vi "PolishVisionV2.vi"() -> (0 "Vison Status":bool, 3 "Image Out":T1)   [LabVIEW 2015]
uses:
  <vilib>/vision/Image Controls.llb/IMAQ Image.ctl
  <vilib>/userdefined/High Color/IMAQdx.ctl
  <vilib>/vision/Pattern Matching.llb/IMAQ Curve Parameters.ctl
  <vilib>/vision/Pattern Matching.llb/IMAQ Match Range Setting.ctl
  <vilib>/vision/driver/NI_Vision_Acquisition_Software.lvlib
  <vilib>/vision/NI_Vision_Development_Module.lvlib
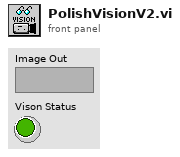
[diagram p1: front panel]
types:
  T1 = typedef "IMAQ Image.ctl" = refnum<image>
  T2 = typedef "IMAQdx.ctl" = refnum<k21>
  T3 = typedef "Image Type" = u32
  T4 = cluster{"Origin Pixel":cluster{"X":sgl, "Y":sgl}, "X Axis Pixel":cluster{"X":sgl, "Y":sgl}, "Axis Reference":u32}
  T5 = cluster{"Position":cluster{"X":sgl, "Y":sgl}, "Radius":dbl, "Score":dbl}[]
  T6 = cluster{"Circles[0]":cluster{"Position":cluster{"X":sgl, "Y":sgl}, "Radius":dbl, "Score":dbl}, "Circles[1]":cluster{"Position":cluster{"X":sgl, "Y":sgl}, "Radius":dbl, "Score":dbl}, "Circles[2]":cluster{"Position":cluster{"X":sgl, "Y":sgl}, "Radius":dbl, "Score":dbl}, "Circles[3]":cluster{"Position":cluster{"X":sgl, "Y":sgl}, "Radius":dbl, "Score":dbl}, "Circles[4]":cluster{"Position":cluster{"X":sgl, "Y":sgl}, "Radius":dbl, "Score":dbl}, "Circles[5]":cluster{"Position":cluster{"X":sgl, "Y":sgl}, "Radius":dbl, "Score":dbl}, "Circles[6]":cluster{"Position":cluster{"X":sgl, "Y":sgl}, "Radius":dbl, "Score":dbl}, "Circles[7]":cluster{"Position":cluster{"X":sgl, "Y":sgl}, "Radius":dbl, "Score":dbl}, "Circles[8]":cluster{"Position":cluster{"X":sgl, "Y":sgl}, "Radius":dbl, "Score":dbl}}
  T7 = typedef "IMAQ Curve Parameters.ctl" = cluster{"Extraction Mode":u32, "Edge Threshold":i32, "Edge Filter Size":u32, "Min Length":i32, "Row Search Step Size":i32, "Col Search Step Size":i32, "Max Endpoint Gap":i32, "Closed":bool, "Subpixel":bool}
  T8 = typedef "IMAQ Match Range Setting.ctl" = cluster{"Match Constraints":u32, "Min":dbl, "Max":dbl}
  T9 = cluster{"Curve Parameters":T7, "Match Mode":cluster{"Rotation":bool, "Scale":bool, "Occlusion":bool, "Reserved":bool, "Reserved":bool, "Reserved":bool}, "Range Settings":T8[], "Number of Matches":i32, "Minimum Match Score":sgl, "SubPixel Accuracy":bool, "Adv. Geometric Match Options 2":cluster{"Setup Data Item":u16, "Item Value":dbl}[]}
  T10 = cluster{"Global Rectangle":i32[], "Contours":cluster{"ID":enum32{"External", "Internal"}, "Type":u32, "Coordinates":i32[]}[]}
  T11 = typedef "IMAQ GM Match Report.ctl" = cluster{"Position":cluster{"x":sgl, "y":sgl}, "Angle":sgl, "Scale":sgl, "Score":sgl, "Bounding Box":cluster{"x":sgl, "y":sgl}[], "Contrast Reversed":bool, "Occlusion %":sgl, "Template Target Curve Score":sgl, "Target Template Curve Score":sgl, "Correlation Score":sgl}
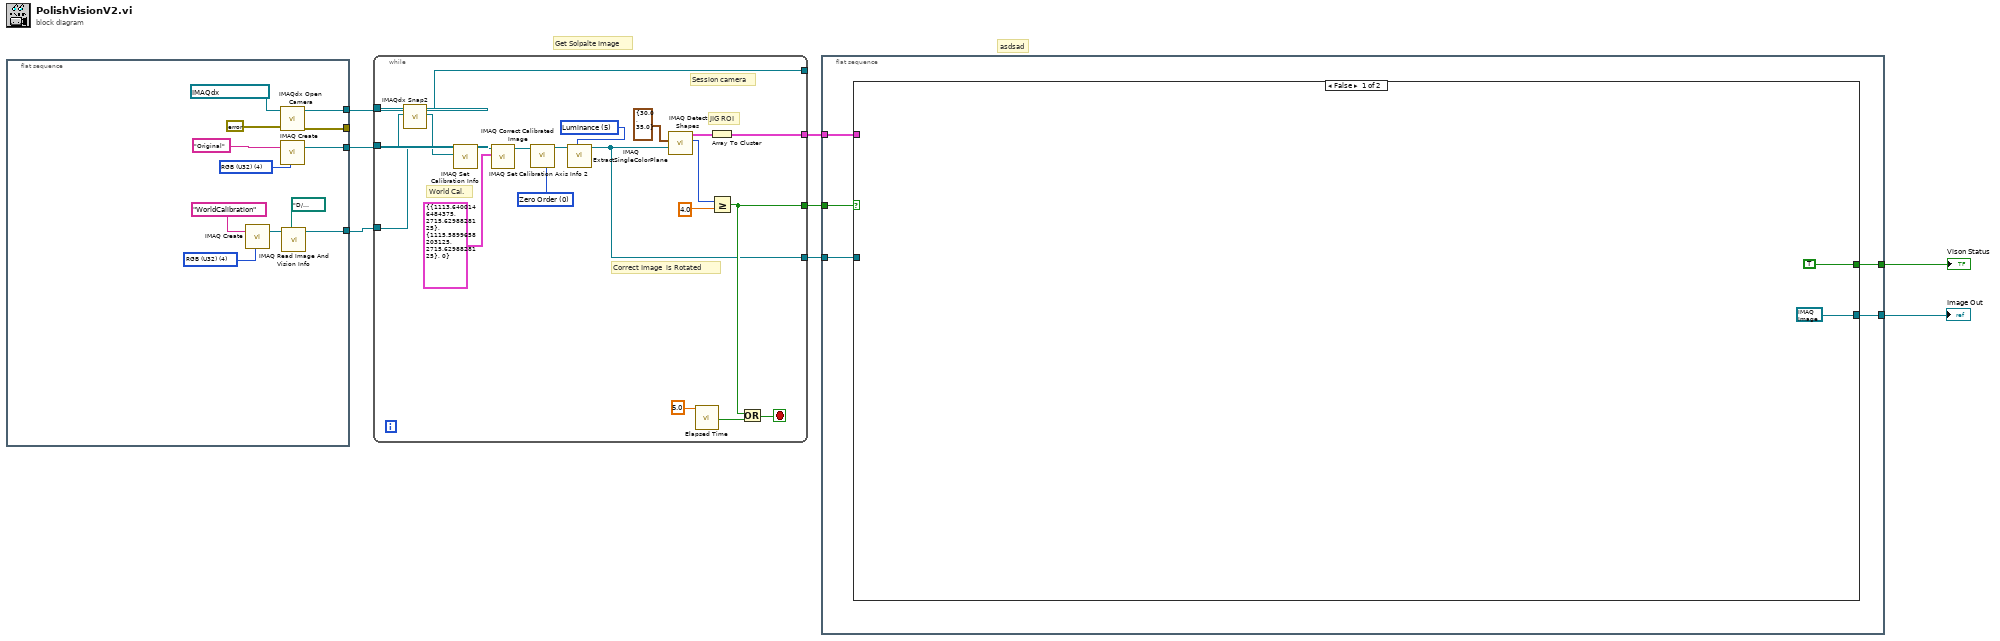
[diagram p0: block diagram]
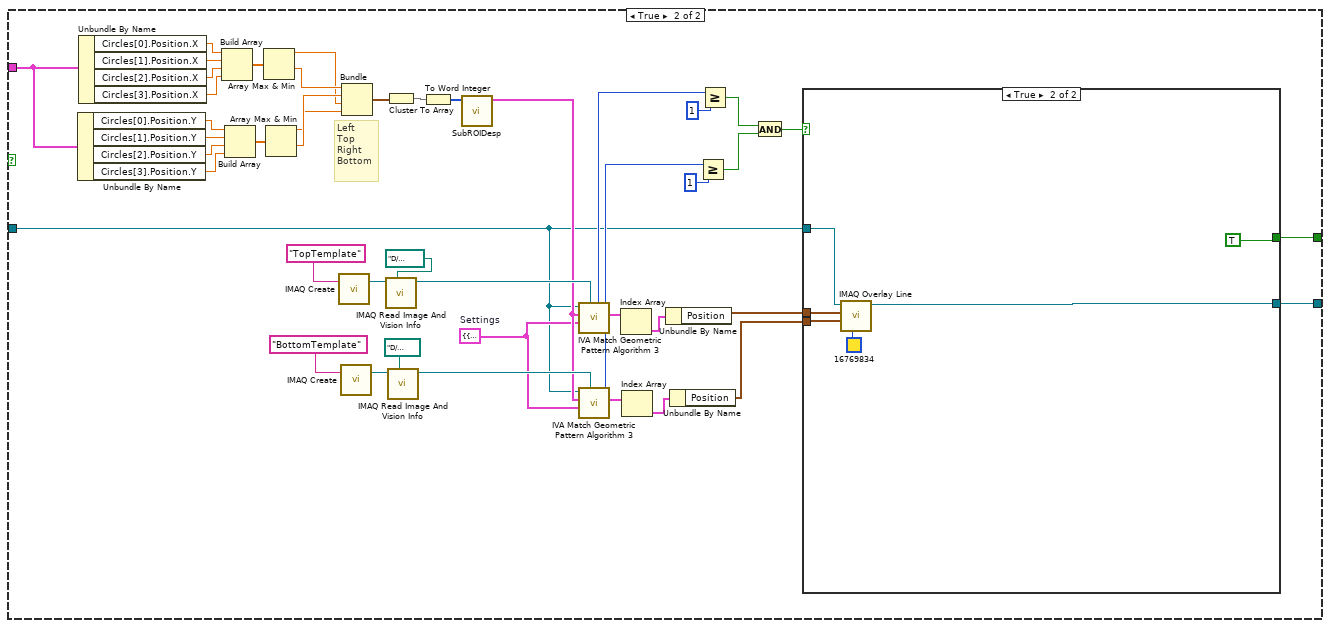
[diagram p2: hidden frame]
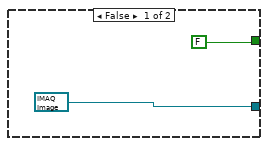
[diagram p3: hidden frame]
diagram:
  # "Get Solpalte Image"
  # "asdsad"
  n1 = flat-sequence {
    tunnel: [w17] -> w8
    tunnel: [w16] -> w7
    tunnel: [w15] -> _
    tunnel: [w10] -> w6
    frame #0 {
      w14 = T3 4 items=["Grayscale (U8)", "Grayscale (I16)", "Grayscale (SGL)", "Complex (CSG)", "RGB (U32)", "HSL (U32)", "RGB (U64)", "Grayscale (U16)"] ("Image Type")
      w18 = T3 4 items=["Grayscale (U8)", "Grayscale (I16)", "Grayscale (SGL)", "Complex (CSG)", "RGB (U32)", "HSL (U32)", "RGB (U64)", "Grayscale (U16)"] ("Image Type")
      n2 = call "IMAQ Create"("Image Name"="WorldCalibration", "Image Type"=w14) -> ("New Image"=w12:T1)  [unwired: 2 in, 2 out]
      n3 = call <vilib>:"IMAQdx Open Camera.vi"("error in"=errorcluster {"status"=FALSE, "code"=0, "source"=""}, "Session In"=T2 "RobotPolishCAM") -> ("error out"=w15:errorcluster, "Session Out"=w17:T2)  [unwired: 8 in]
      n4 = call "IMAQ Create"("Image Name"="Original", "Image Type"=w18) -> ("New Image"=w16:T1)  [unwired: 3 in, 1 out]
      n5 = call "IMAQ Read Image And Vision Info"("File Path"=path "D:/PolishingRobot/LastEdition/config setting/WorldCalV2.png", "Image"=w12) -> ("Image Out"=w10:T1)  [unwired: 2 in, 7 out]
    }
  }
  n6 = while {
    tunnel: w8 -> [w41]
    tunnel: w7 -> [w40]
    tunnel: [w28] -> w5
    tunnel: [w34] -> _
    tunnel: w6 -> [w22]
    tunnel: [w24] -> w4
    tunnel: [w23] -> w3
    stop <- w25 stop-if-true
    w31 = u32 0 items=["Zero Order", "Bi-Linear", "Quadratic", "Cubic Spline"] ("Interpolation Type")
    w39 = 5 items=["Red", "Green", "Blue", "Hue", "Saturation", "Luminance", "Value", "Intensity"] ("Color Plane")
    # "Correct Image  is Rotated"
    # "Session camera"
    # "World Cal."
    # "JIG ROI"
    n7 = call <vilib>:"IMAQdx Snap2.vi"("Image In"=w40, "Session In"=w41) -> ("Image Out"=w21:T1, "Session Out"=w34:T2)  [unwired: 7 in, 1 out]
    n8 = call "IMAQ Set Calibration Info"("Image Dst"=w21, "Image Src"=w22) -> ("Calibrated Image"=w32:T1)  [unwired: 2 in, 7 out]
    n9 = call-poly "IMAQ Set Calibration Axis Info 2"("Calibration Axis Info"=T4 {"Origin Pixel"={"X"=1113.64, "Y"=2715.63}, "X Axis Pixel"={"X"=1115.59, "Y"=2715.63}, "Axis Reference"=0}, "Calibration Template Image In"=w32) -> ("Calibration Template Image Out"=w30:T1)  [unwired: 1 in, 8 out]
    n10 = call "IMAQ Correct Calibrated Image"("Interpolation Type"=w31, "Image Src"=w30) -> ("Corrected Image"=w29:T1)  [unwired: 5 in, 4 out]
    n11 = call "IMAQ ExtractSingleColorPlane"("Color Plane"=w39, "Image Src"=w29) -> ("Image Dst Out"=w23:T1)  [unwired: 8 in, 1 out]
    n12 = call-poly "IMAQ Detect Shapes"("Circle Descriptor"=cluster{"Min Radius":dbl, "Max Radius":dbl} {"Min Radius"=30.0, "Max Radius"=35.0}, "Image"=w23) -> ("Number of Matches Returned"=w35:i32, "Circles"=w36:T5)  [unwired: 7 in, 1 out]
    n13 = call "Elapsed Time"("Time Target (s)"=5.0) -> ("Time has Elapsed"=w26:bool)  [unwired: 11 in, 7 out]
    n14 = Array To Cluster(array=w36) -> (cluster=w28:T6)
    n15 = Greater Or Equal?(x=w35, y=4.0) -> (x >= y?=w24:bool)
    n16 = Or(x=w24, y=w26) -> (x .or. y?=w25:bool)
  }
  n17 = flat-sequence {
    tunnel: w5 -> [w44]
    tunnel: w4 -> [w46]
    tunnel: w3 -> [w45]
    tunnel: [w43] -> w2
    tunnel: [w42] -> w1
    frame #0 {
      n18 = case shown="False" w46 {
        tunnel: w45 -> [_ w51]
        tunnel: w44 -> [_ w75]
        tunnel: [T1 refnum ("Image Out 2") w50] -> w43
        tunnel: [TRUE w49] -> w42
        frame False {
        }
        frame True {
          w65 = T9 {"Curve Parameters"={"Extraction Mode"=0, "Edge Threshold"=80, "Edge Filter Size"=1, "Min Length"=30, "Row Search Step Size"=10, "Col Search Step Size"=10, "Max Endpoint Gap"=10, "Closed"=FALSE, "Subpixel"=FALSE}, "Match Mode"={"Rotation"=TRUE, "Scale"=FALSE, "Occlusion"=FALSE, "Reserved"=FALSE, "Reserved"=FALSE, "Reserved"=FALSE}, "Range Settings"=[{"Match Constraints"=0, "Min"=-10.0, "Max"=10.0}], "Number of Matches"=1, "Minimum Match Score"=800.0, "SubPixel Accuracy"=FALSE, "Adv. Geometric Match Options 2"=[{"Setup Data Item"=21, "Item Value"=0.0}, {"Setup Data Item"=22, "Item Value"=1.0}]}  # Settings
          # "Left \nTop\nRight \nBottom"
          n19 = Unbundle By Name(w75) -> ("Circles[0].Position.Y"=w80:sgl, "Circles[1].Position.Y"=w79:sgl, "Circles[2].Position.Y"=w78:sgl, "Circles[3].Position.Y"=w77:sgl)
          n20 = Unbundle By Name(w75) -> ("Circles[0].Position.X"=w84:sgl, "Circles[1].Position.X"=w83:sgl, "Circles[2].Position.X"=w82:sgl, "Circles[3].Position.X"=w81:sgl)
          n21 = Build Array(w84, w83, w82, w81) -> (w76:sgl[])
          n22 = Build Array(w80, w79, w78, w77) -> (w74:sgl[])
          n23 = Array Max & Min(array=w76) -> (max value=w71:sgl, min value=w73:sgl)  [unwired: 2 out]
          n24 = Array Max & Min(array=w74) -> (max value=w70:sgl, min value=w72:sgl)  [unwired: 2 out]
          n25 = call "IMAQ Create"("Image Name"="TopTemplate") -> ("New Image"=w91:T1)  [unwired: 3 in, 2 out]
          n26 = call "IMAQ Create"("Image Name"="BottomTemplate") -> ("New Image"=w89:T1)  [unwired: 3 in, 2 out]
          n27 = Bundle(w73, w72, w71, w70) -> (w69:cluster{sgl, sgl, sgl, sgl})  [unwired: 1 in]
          n28 = Cluster To Array(cluster=w69) -> (array=w68:sgl[])
          n29 = call "IMAQ Read Image And Vision Info"("File Path"=path "D:/PolishingRobot/LastEdition/config setting/geomath/Top.png" ("Template File Path"), "Image"=w91) -> ("Image Out"=w86:T1)  [unwired: 2 in, 7 out]
          n30 = call "IMAQ Read Image And Vision Info"("File Path"=path "D:/PolishingRobot/LastEdition/config setting/geomath/bottom.png", "Image"=w89) -> ("Image Out"=w85:T1)  [unwired: 2 in, 7 out]
          n31 = To Word Integer(number=w68) -> (16bit integer=w67:i16[])
          n32 = call "SubROIDesp.vi"("Array"=w67) -> ("output cluster"=w66:T10)  [unwired: 10 in]
          n33 = call <vilib>:"IVA Match Geometric Pattern Algorithm 3.vi"("Template"=w86, "Settings"=w65, "ROI Descriptor"=w66, "Image"=w51) -> ("Matches"=w56:T11[], "Number of Matches"=w64:i32)  [unwired: 1 in, 5 out]
          n34 = call <vilib>:"IVA Match Geometric Pattern Algorithm 3.vi"("Template"=w85, "Settings"=w65, "ROI Descriptor"=w66, "Image"=w51) -> ("Matches"=w58:T11[], "Number of Matches"=w61:i32)  [unwired: 1 in, 5 out]
          n35 = Index Array(array=w56) -> (element=w57:T11)  [unwired: 1 in]
          n36 = Index Array(array=w58) -> (element=w53:T11)  [unwired: 1 in]
          n37 = Unbundle By Name(w57) -> ("Position"=w54:cluster{"x":sgl, "y":sgl})
          n38 = Unbundle By Name(w53) -> ("Position"=w52:cluster{"x":sgl, "y":sgl})
          n39 = Greater Or Equal?(x=w61, y=1) -> (x >= y?=w59:bool)
          n40 = Greater Or Equal?(x=w64, y=1) -> (x >= y?=w60:bool)
          n41 = And(x=w60, y=w59) -> (x .and. y?=w55:bool)
          n42 = case shown="True" w55 {
            tunnel: w54 -> [_ w100]
            tunnel: w52 -> [_ w99]
            tunnel: w51 -> [_ w98]
            tunnel: [T1 refnum ("Image Out 2") w96] -> w50
            tunnel: [FALSE TRUE] -> w49
            frame False {
            }
            frame True {
              n43 = call "IMAQ Overlay Line"("Color"=u32 16769834, "End Point"=w99, "Start Point"=w100, "Image"=w98) -> ("Image Out"=w96:T1)  [unwired: 6 in, 1 out]
            }
          }
        }
      }
    }
  }
  "Image Out" <- w2
  "Vison Status" <- w1
